vi "get_argument_types.vi"(8 "error in (no error)":errorcluster, 11 "FunctionType in":refnum<class "FunctionType.lvclass">) -> (0 "error out":errorcluster, 2 "argument_types":refnum<class "Type.lvclass">[](array[class]), 3 "FunctionType out":refnum<class "FunctionType.lvclass">)   [LabVIEW 2020, in "mlir.lvlib" / "FunctionType.lvclass"]
uses:
  FunctionType.lvclass
  FunctionType.lvclass/FunctionType.ctl
  Type/Type.lvclass
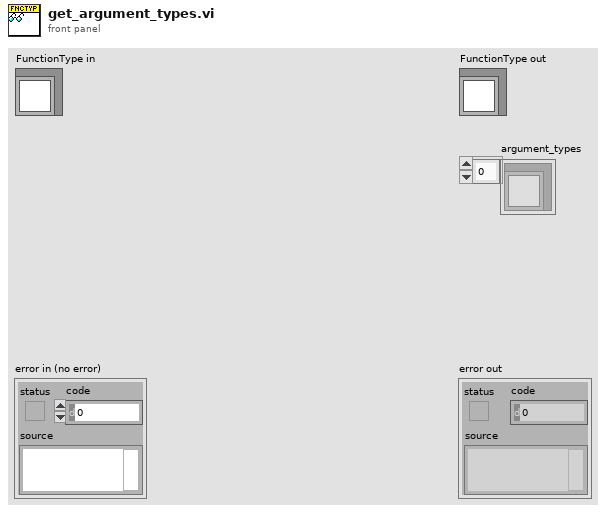
[diagram p1: front panel]
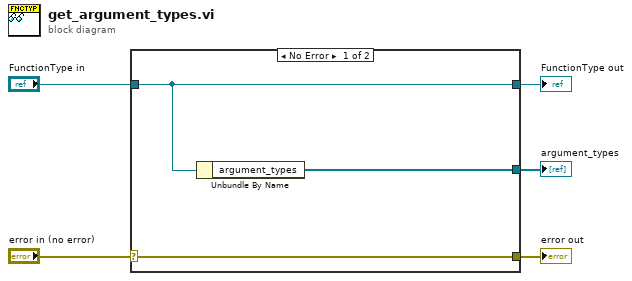
[diagram p0: block diagram]
diagram:
  n1 = case shown="No Error" "error in (no error)" {
    selector: "error in (no error)" -> [w8 w9]
    tunnel: [w8 w9] -> w4
    tunnel: [w7 w10] -> w2
    tunnel: "FunctionType in" -> [w7 w10]
    tunnel: [w6 _] -> w1
    frame No Error {
      n2 = Unbundle By Name(w7) -> ("argument_types"=w6:refnum<class "Type.lvclass">[])
    }
    frame Error {
    }
  }
  "error out" <- w4
  "FunctionType out" <- w2
  "argument_types" <- w1
